vi "保持寄存器解析.vi"(11 "A读保持寄存器信息组":T2(array[cluster])=[{"地址"=10099, "数量"=2, "寄存器值"=[0, 0], "名称"="产品总数"}, {"地址"=10101, "数量"=2, "寄存器值"=[0, 0], "名称"="合格数量"}, {"地址"=10103, "数量"=2, "寄存器值"=[0, 0], "名称"="泄露数量"}, {"地址"=506, "数量"=2, "寄存器值"=[0, 0], "名称"="1测试时间"}, {"地址"=508, "数量"=2, "寄存器值"=[0, 0], "名称"="1测试泄漏"}, {"地址"=1506, "数量"=2, "寄存器值"=[0, 0], "名称"="2测试时间"}, {"地址"=1508, "数量"=2, "寄存器值"=[0, 0], "名称"="2采样泄漏"}, {"地址"=504, "数量"=2, "寄存器值"=[0, 0], "名称"="1#目标压力"}, {"地址"=498, "数量"=1, "寄存器值"=[0, 0], "名称"="1#测试结果"}, {"地址"=1498, "数量"=1, "寄存器值"=[0, 64], "名称"="2#测试结果"}, {"地址"=1504, "数量"=2, "寄存器值"=[0, 0], "名称"="2#目标压力"}, {"地址"=500, "数量"=1, "寄存器值"=[0], "名称"="实时压力"}] {"寄存器值" format="%x"}) -> (2 "运行状态":string, 3 "参数值":T1(array[cluster]))   [LabVIEW 2015]
panel:
  out "参数组别":u32
  out "测试时间":dbl
  out "参数值":string[](array[string])
  out "失败原因":string
  out "1OK":bool
  out "测试结果  1":string
  out "门限压力":i32
  out "实时压力":i32
  out "目标压力":i32
  out "泄漏压力":dbl
  out "NG":u32
  out "OK":u32
  out "总量":u32
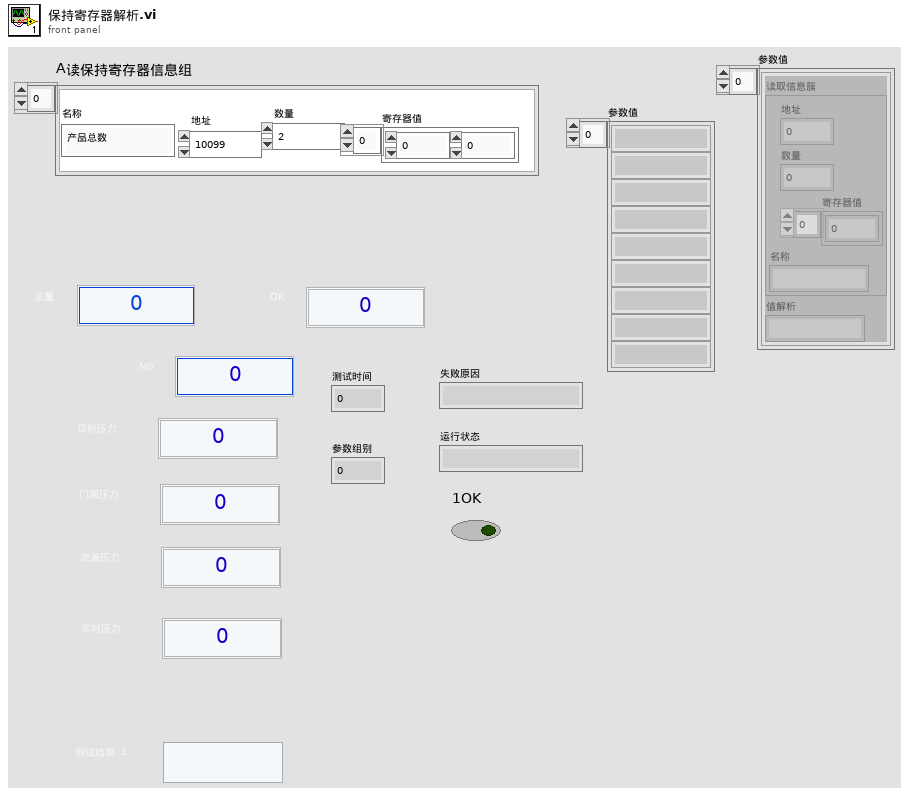
[diagram p1: front panel]
types:
  T1 = cluster{"读取信息簇":cluster{"地址":u16, "数量":u16, "寄存器值":u16[], "名称":string}, "值解析":string}[]
  T2 = cluster{"地址":u16, "数量":u16, "寄存器值":u16[], "名称":string}[]
  T3 = cluster{"读取信息簇":cluster{"地址":u16, "数量":u16, "寄存器值":u16[], "名称":string}, "值解析":string}
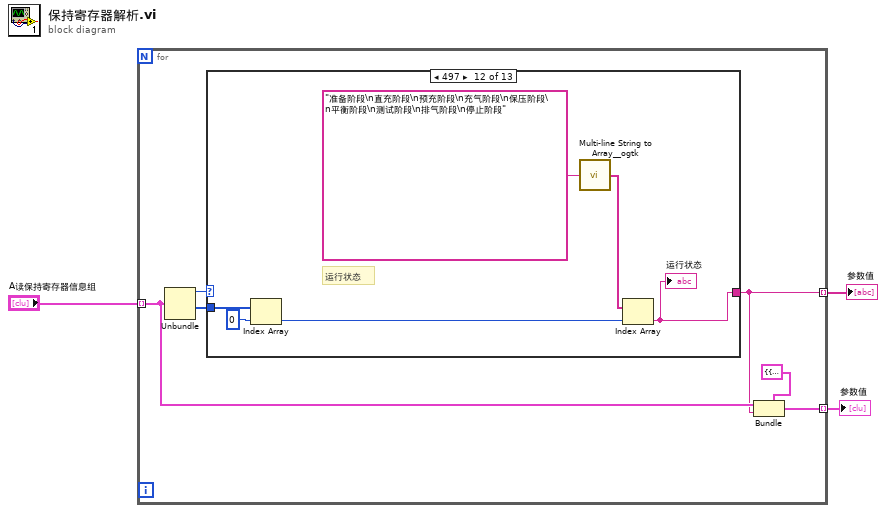
[diagram p0: block diagram]
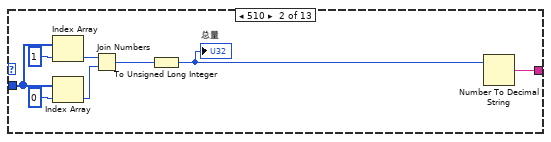
[diagram p3: hidden frame]
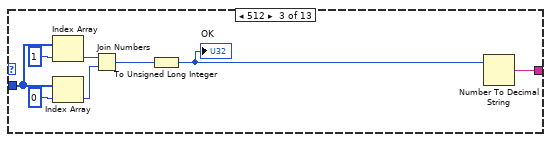
[diagram p4: hidden frame]
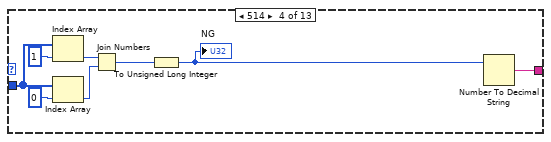
[diagram p5: hidden frame]
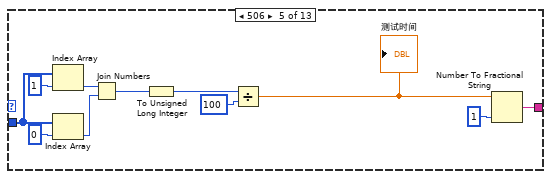
[diagram p6: hidden frame]
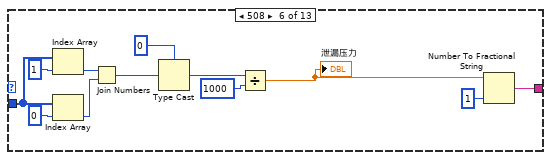
[diagram p7: hidden frame]
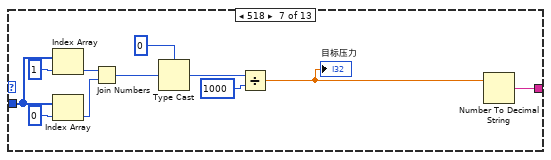
[diagram p8: hidden frame]
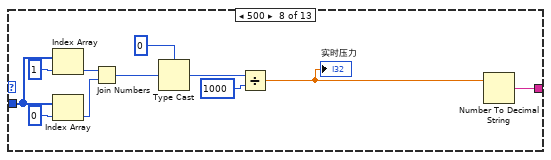
[diagram p9: hidden frame]
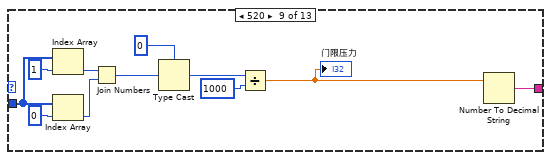
[diagram p10: hidden frame]
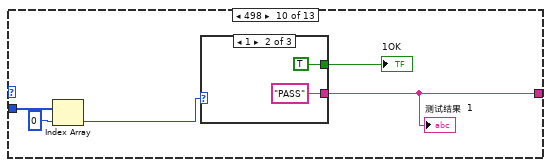
[diagram p11: hidden frame]
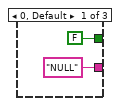
[diagram p12: hidden frame]
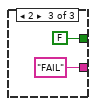
[diagram p13: hidden frame]
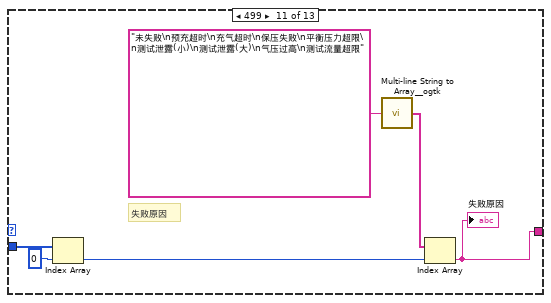
[diagram p14: hidden frame]
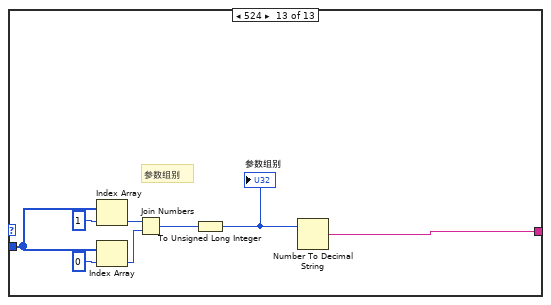
[diagram p15: hidden frame]
diagram:
  n1 = for {
    tunnel: "A读保持寄存器信息组" -> [w7] mode=indexing
    tunnel: [w6] -> w2 mode=indexing
    tunnel: [w5] -> w1 mode=indexing
    n2 = Unbundle(w7) -> ("地址"=w9:u16, "寄存器值"=w8:u16[])  [unwired: 2 out]
    n3 = case shown="497" w9 {
      tunnel: w8 -> [_ w16 w24 w32 w43 w55 w61 w72 w83 w93 w105 w111 w115]
      tunnel: [_ w10 w18 w26 w34 w47 w57 w68 w79 w90 w101 w107 w114] -> w6
      frame Default {
      }
      frame 510 {
        n4 = Index Array(array=w16, index=1 ("索引")) -> (element=w14:u16)
        n5 = Index Array(array=w16, index=0 ("索引")) -> (element=w13:u16)
        n6 = Join Numbers(hi=w14, lo=w13) -> ((hi.lo)=w12:u32)
        n7 = To Unsigned Long Integer(number=w12) -> (unsigned 32bit integer=w11:u32)
        "总量" <- w11
        n8 = Number To Decimal String(number=w11) -> (decimal integer string=w10:string)  [unwired: 1 in]
      }
      frame 512 {
        n9 = Index Array(array=w24, index=1 ("索引")) -> (element=w22:u16)
        n10 = Index Array(array=w24, index=0 ("索引")) -> (element=w21:u16)
        n11 = Join Numbers(hi=w22, lo=w21) -> ((hi.lo)=w20:u32)
        n12 = To Unsigned Long Integer(number=w20) -> (unsigned 32bit integer=w19:u32)
        "OK" <- w19
        n13 = Number To Decimal String(number=w19) -> (decimal integer string=w18:string)  [unwired: 1 in]
      }
      frame 514 {
        n14 = Index Array(array=w32, index=1 ("索引")) -> (element=w30:u16)
        n15 = Index Array(array=w32, index=0 ("索引")) -> (element=w29:u16)
        n16 = Join Numbers(hi=w30, lo=w29) -> ((hi.lo)=w28:u32)
        n17 = To Unsigned Long Integer(number=w28) -> (unsigned 32bit integer=w27:u32)
        "NG" <- w27
        n18 = Number To Decimal String(number=w27) -> (decimal integer string=w26:string)  [unwired: 1 in]
      }
      frame 506 {
        n19 = Index Array(array=w43, index=1 ("索引")) -> (element=w41:u16)
        n20 = Index Array(array=w43, index=0 ("索引")) -> (element=w40:u16)
        n21 = Join Numbers(hi=w41, lo=w40) -> ((hi.lo)=w39:u32)
        n22 = To Unsigned Long Integer(number=w39) -> (unsigned 32bit integer=w38:u32)
        n23 = Divide(x=w38, y=u32 100) -> (x/y=w36:dbl)
        "测试时间" <- w36
        n24 = Number To Fractional String(number=w36, precision (6)=i16 1 ("精度(6)")) -> (F-format string=w34:string)  [unwired: 2 in]
      }
      frame 508 {
        n25 = Index Array(array=w55, index=1 ("索引")) -> (element=w53:u16)
        n26 = Index Array(array=w55, index=0 ("索引")) -> (element=w52:u16)
        n27 = Join Numbers(hi=w53, lo=w52) -> ((hi.lo)=w51:u32)
        n28 = Type Cast(type=0 ("泄漏压力"), x=w51) -> (*(type *) &x=w48:i32)
        n29 = Divide(x=w48, y=u32 1000) -> (x/y=w46:dbl)
        "泄漏压力" <- w46
        n30 = Number To Fractional String(number=w46, precision (6)=i16 1 ("精度(6)")) -> (F-format string=w47:string)  [unwired: 2 in]
      }
      frame 518 {
        n31 = Index Array(array=w61, index=1 ("索引")) -> (element=w67:u16)
        n32 = Index Array(array=w61, index=0 ("索引")) -> (element=w66:u16)
        n33 = Join Numbers(hi=w67, lo=w66) -> ((hi.lo)=w65:u32)
        n34 = Type Cast(type=0 ("泄漏压力"), x=w65) -> (*(type *) &x=w59:i32)
        n35 = Divide(x=w59, y=u32 1000) -> (x/y=w58:dbl)
        "目标压力" <- w58
        n36 = Number To Decimal String(number=w58) -> (decimal integer string=w57:string)  [unwired: 1 in]
      }
      frame 500 {
        n37 = Index Array(array=w72, index=1 ("索引")) -> (element=w78:u16)
        n38 = Index Array(array=w72, index=0 ("索引")) -> (element=w77:u16)
        n39 = Join Numbers(hi=w78, lo=w77) -> ((hi.lo)=w76:u32)
        n40 = Type Cast(type=0 ("泄漏压力"), x=w76) -> (*(type *) &x=w70:i32)
        n41 = Divide(x=w70, y=u32 1000) -> (x/y=w69:dbl)
        "实时压力" <- w69
        n42 = Number To Decimal String(number=w69) -> (decimal integer string=w68:string)  [unwired: 1 in]
      }
      frame 520 {
        n43 = Index Array(array=w83, index=1 ("索引")) -> (element=w89:u16)
        n44 = Index Array(array=w83, index=0 ("索引")) -> (element=w88:u16)
        n45 = Join Numbers(hi=w89, lo=w88) -> ((hi.lo)=w87:u32)
        n46 = Type Cast(type=0 ("泄漏压力"), x=w87) -> (*(type *) &x=w81:i32)
        n47 = Divide(x=w81, y=u32 1000) -> (x/y=w80:dbl)
        "门限压力" <- w80
        n48 = Number To Decimal String(number=w80) -> (decimal integer string=w79:string)  [unwired: 1 in]
      }
      frame 498 {
        n49 = Index Array(array=w93, index=0 ("索引")) -> (element=w91:u16)
        n50 = case shown="1" w91 {
          tunnel: [FALSE ("1OK") TRUE ("1OK") FALSE ("1OK")] -> w92
          tunnel: ["NULL" ("格式字符串") "PASS" ("格式字符串") "FAIL" ("格式字符串")] -> w90
          frame 0, Default {
          }
          frame 1 {
          }
          frame 2 {
          }
        }
        "1OK" <- w92
        "测试结果  1" <- w90
      }
      frame 499 {
        # "失败原因"
        n51 = Index Array(array=w105, index=0 ("索引")) -> (element=w102:u16)
        n52 = call <userlib>:"Multi-line String to Array__ogtk.vi"("string"="未失败\n预充超时\n充气超时\n保压失败\n平衡压力超限\n测试泄露(小)\n测试泄露(大)\n气压过高\n测试流量超限") -> ("lines"=w103:string[])
        n53 = Index Array(array=w103, index=w102) -> (element=w101:string)
        "失败原因" <- w101
      }
      frame 497 {
        # "运行状态"
        n54 = Index Array(array=w111, index=0 ("索引")) -> (element=w108:u16)
        n55 = call <userlib>:"Multi-line String to Array__ogtk.vi"("string"="准备阶段\n直充阶段\n预充阶段\n充气阶段\n保压阶段\n平衡阶段\n测试阶段\n排气阶段\n停止阶段") -> ("lines"=w109:string[])
        n56 = Index Array(array=w109, index=w108) -> (element=w107:string)
        "运行状态" <- w107
      }
      frame 524 {
        # "参数组别"
        n57 = Index Array(array=w115, index=1 ("索引")) -> (element=w118:u16)
        n58 = Index Array(array=w115, index=0 ("索引")) -> (element=w117:u16)
        n59 = Join Numbers(hi=w118, lo=w117) -> ((hi.lo)=w116:u32)
        n60 = To Unsigned Long Integer(number=w116) -> (unsigned 32bit integer=w113:u32)
        "参数组别" <- w113
        n61 = Number To Decimal String(number=w113) -> (decimal integer string=w114:string)  [unwired: 1 in]
      }
    }
    n62 = Bundle(cluster=T3 {"读取信息簇"={"地址"=0, "数量"=0, "寄存器值"=[], "名称"=""}, "值解析"=""} ("簇"), "读取信息簇"=w7, "值解析"=w6) -> (w5:T3)
  }
  "参数值" <- w2
  "参数值" <- w1
